vi "21b calculate.vi"(11 "Data":T2) -> (3 "Data Out":T2)   [LabVIEW 2020]
uses:
  Problem-21/ENUM_Operator.ctl
  Problem-21/Cluster 21b_Monkey Data.ctl
panel:
  out "Operator":T1
  out "2":i64
  out "1":i64
  out "value":i64
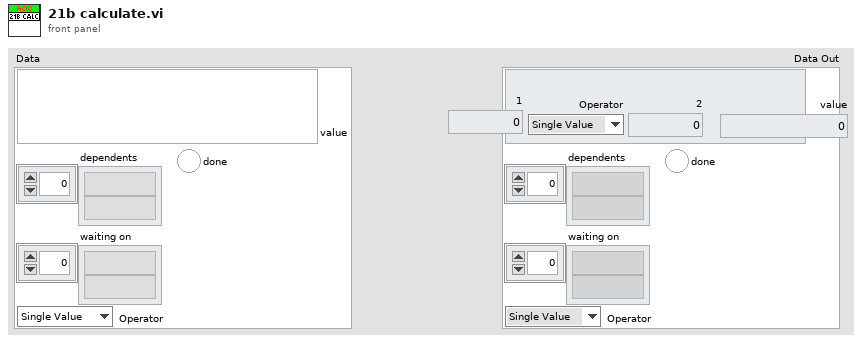
[diagram p1: front panel]
types:
  T1 = typedef "ENUM_Operator.ctl" = enum16{"Single Value", "Add", "Subtract", "Multiply", "Divide"}
  T2 = typedef "Cluster 21b_Monkey Data.ctl" = cluster{"done":bool, "value":string, "dependents":string[], "waiting on":string[], "Operator":T1}
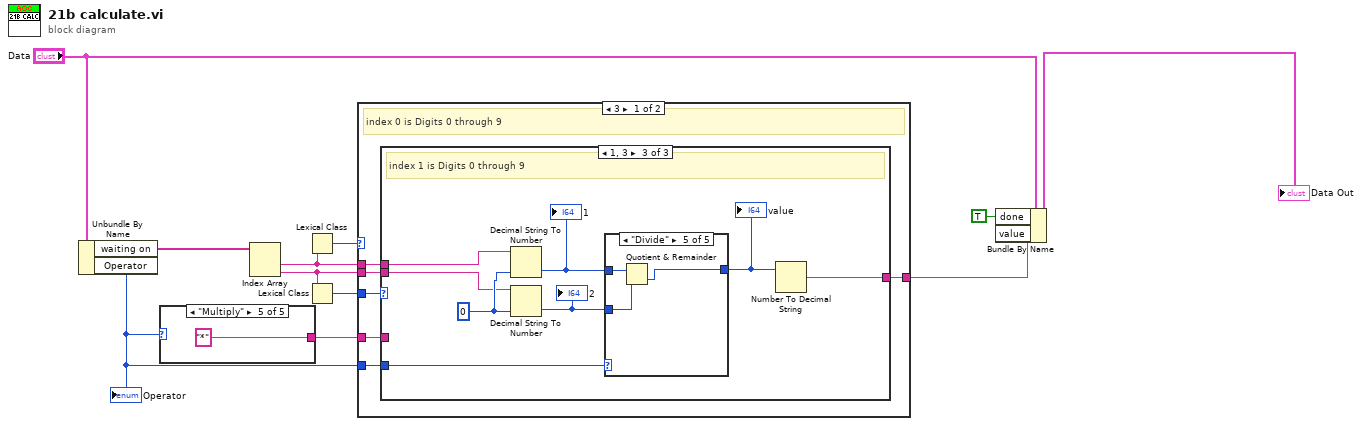
[diagram p0: block diagram]
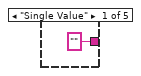
[diagram p2: hidden frame]
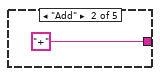
[diagram p3: hidden frame]
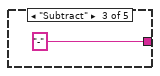
[diagram p4: hidden frame]
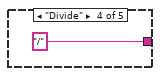
[diagram p5: hidden frame]
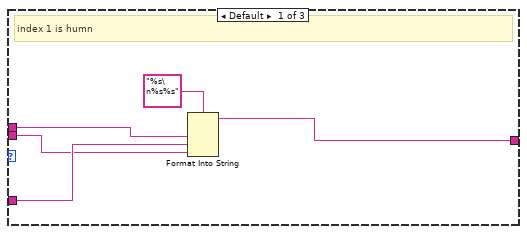
[diagram p6: hidden frame]
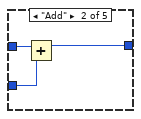
[diagram p9: hidden frame]
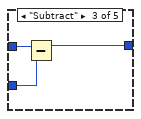
[diagram p10: hidden frame]
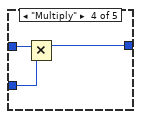
[diagram p11: hidden frame]
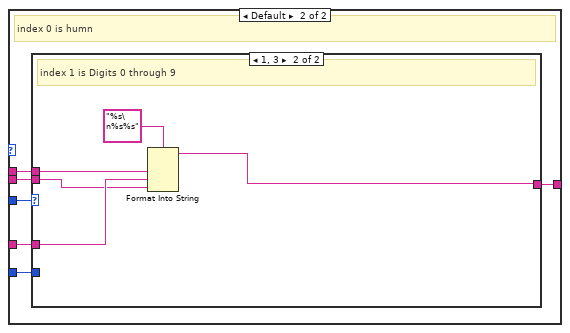
[diagram p12: hidden frame]
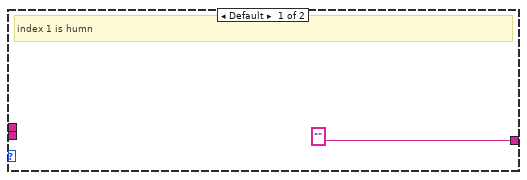
[diagram p13: hidden frame]
diagram:
  n1 = Unbundle By Name("Data") -> ("waiting on"=w8:string[], "Operator"=w2:T1)
  "Operator" <- w2
  n2 = case shown="\"Multiply\"" w2 {
    tunnel: ["" "+" "-" "/" "*"] -> w1
    frame "Single Value" {
    }
    frame "Add" {
    }
    frame "Subtract" {
    }
    frame "Divide" {
    }
    frame "Multiply" {
    }
  }
  n3 = Index Array(array=w8) -> (element #1=w7:string, element #2=w6:string)  [unwired: 2 in]
  n4 = Lexical Class(1:w7) -> (0:w5:i16)
  n5 = Lexical Class(1:w6) -> (0:w4:i16)
  n6 = case shown="3" w5 {
    tunnel: w2 -> [w22 w54]
    tunnel: w7 -> [w21 w53]
    tunnel: w6 -> [w20 w52]
    tunnel: w4 -> [w19 w51]
    tunnel: [w18 w50] -> w3
    tunnel: w1 -> [w17 w49]
    frame 3 {
      # "index 0 is Digits 0 through 9"
      n7 = case shown="1, 3" w19 {
        tunnel: w22 -> [_ _ w35]
        tunnel: w21 -> [w26 _ w31]
        tunnel: w20 -> [w24 _ w30]
        tunnel: [w23 _ w28] -> w18
        tunnel: w17 -> [w25 _ _]
        frame Default {
          # "index 1 is humn"
          n8 = Format Into String(format string="%s\n%s%s", w26, w25, w24) -> (resulting string=w23:string)  [unwired: 2 in, 1 out]
        }
        frame 1 {
          # "Blank"
        }
        frame 1, 3 {
          w34 = i64 0
          # "index 1 is Digits 0 through 9"
          n9 = Decimal String To Number(string=w31, default (0L)=w34) -> (number=w33:i64)  [unwired: 1 in, 1 out]
          "1" <- w33
          n10 = Decimal String To Number(string=w30, default (0L)=w34) -> (number=w32:i64)  [unwired: 1 in, 1 out]
          "2" <- w32
          n11 = case shown="\"Divide\"" w35 {
            tunnel: w33 -> [w36 w39 w42 w45 w48]
            tunnel: w32 -> [_ w38 w41 w44 w47]
            tunnel: [w36 w37 w40 w43 w46] -> w29
            frame "Single Value" {
            }
            frame "Add" {
              n12 = Add(x=w39, y=w38) -> (x+y=w37:i64)
            }
            frame "Subtract" {
              n13 = Subtract(x=w42, y=w41) -> (x-y=w40:i64)
            }
            frame "Multiply" {
              n14 = Multiply(x=w45, y=w44) -> (x*y=w43:i64)
            }
            frame "Divide" {
              n15 = Quotient & Remainder(x=w48, y=w47) -> (floor(x/y)=w46:i64)  [unwired: 1 out]
            }
          }
          "value" <- w29
          n16 = Number To Decimal String(number=w29) -> (decimal integer string=w28:string)  [unwired: 1 in]
        }
      }
    }
    frame Default {
      # "index 0 is humn"
      n17 = case shown="1, 3" w51 {
        tunnel: w54 -> [_ _]
        tunnel: w53 -> [_ w59]
        tunnel: w52 -> [_ w57]
        tunnel: ["" w56] -> w50
        tunnel: w49 -> [_ w58]
        frame Default {
          # "index 1 is humn"
        }
        frame 1, 3 {
          # "index 1 is Digits 0 through 9"
          n18 = Format Into String(format string="%s\n%s%s", w59, w58, w57) -> (resulting string=w56:string)  [unwired: 2 in, 1 out]
        }
      }
    }
  }
  n19 = Bundle By Name(cluster="Data", "done"=TRUE, "value"=w3) -> (→"Data Out":T2)
